vi "PH_USB600x_AnalogReader.evt call set Prdc Interval.vi"(0 "i ref in":refnum<vi>, 2 "Instance":string, 3 "Prdc Interval [s]":dbl, 5 "error in":errorcluster) -> (14 "i ref out":refnum<vi>, 19 "error out":errorcluster)   [LabVIEW 2014, in "PH_USB600x_AnalogReader.lvlib"]
doc: "This VI sends a simple event call."
uses:
  PH_USB600x_AnalogReader.lvlib
  CSCore/CSSystem/CoreLib/CoreLib.double 2 byte array.vi
  CSCore/BaseProcess/BaseProcess.lvlib
  CSCore/CSSystem/CoreLib/CoreLib.lvlib
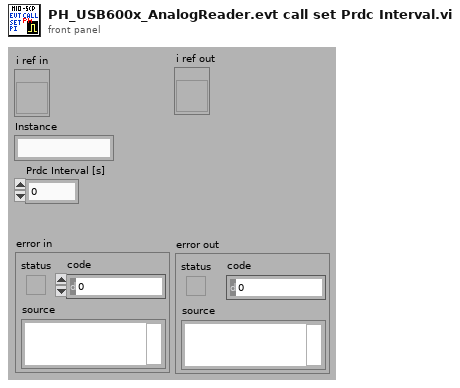
[diagram p1: front panel]
types:
  T1 = typedef "CoreDefs.rawDataType.ctl" = i8[]
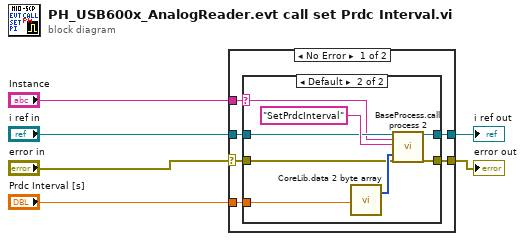
[diagram p0: block diagram]
diagram:
  n1 = case shown="No Error" "error in" {
    selector: "error in" -> [w8 w23]
    tunnel: "Instance" -> [w7 _]
    tunnel: "i ref in" -> [w12 w24]
    tunnel: "Prdc Interval [s]" -> [w11 _]
    tunnel: [w10 w24] -> w4
    tunnel: [w9 w23] -> w3
    frame No Error {
      n2 = case shown="Default" w7 {
        selector: w7 -> [_ w15]
        tunnel: w12 -> [w13 w21]
        tunnel: w11 -> [_ w19]
        tunnel: [w13 w18] -> w10
        tunnel: [w14 w17] -> w9
        tunnel: w8 -> [w14 w16]
        frame "", "N/A" {
        }
        frame Default {
          n3 = call-poly "CoreLib.data 2 byte array.vi"("f64"=w19) -> ("byteArray out"=w20:T1)  [unwired: 18 in]
          n4 = call "BaseProcess.call process 2.vi"("i ref in"=w21, "Object"=w15, "Selector"="SetPrdcInterval", "Data"=w20, "error in (no error)"=w16) -> ("i ref out"=w18:refnum<vi>, "error out"=w17:errorcluster)  [unwired: 13 in]
        }
      }
    }
    frame Error {
    }
  }
  "i ref out" <- w4
  "error out" <- w3
